vi "Host_17.vi"() -> ()   [LabVIEW 2017]
panel:
  in  "stop":bool
  out "Motor Speed":cluster{i32, dbl}[](graph)
  out "Armature Current":cluster{i32, dbl}[](graph)
  out "Feedback Load Torque 2":dbl
  out "Feedback Duty Cycle 2":dbl
  in  "Duty Cycle 2":dbl(slide) scale=0.0..100.0
  in  "Load Torque 2":dbl(slide) scale=-0.2..0.2
  in  "Data Update Speed (ms)":dbl
  in  "Website Button":bool
  in  "Doc Button":bool
  in  "Save Button":bool
  in  "Run Button":bool
  # "OPAL-RT Real Time Outputs"
  # "Microcontroller Inputs"
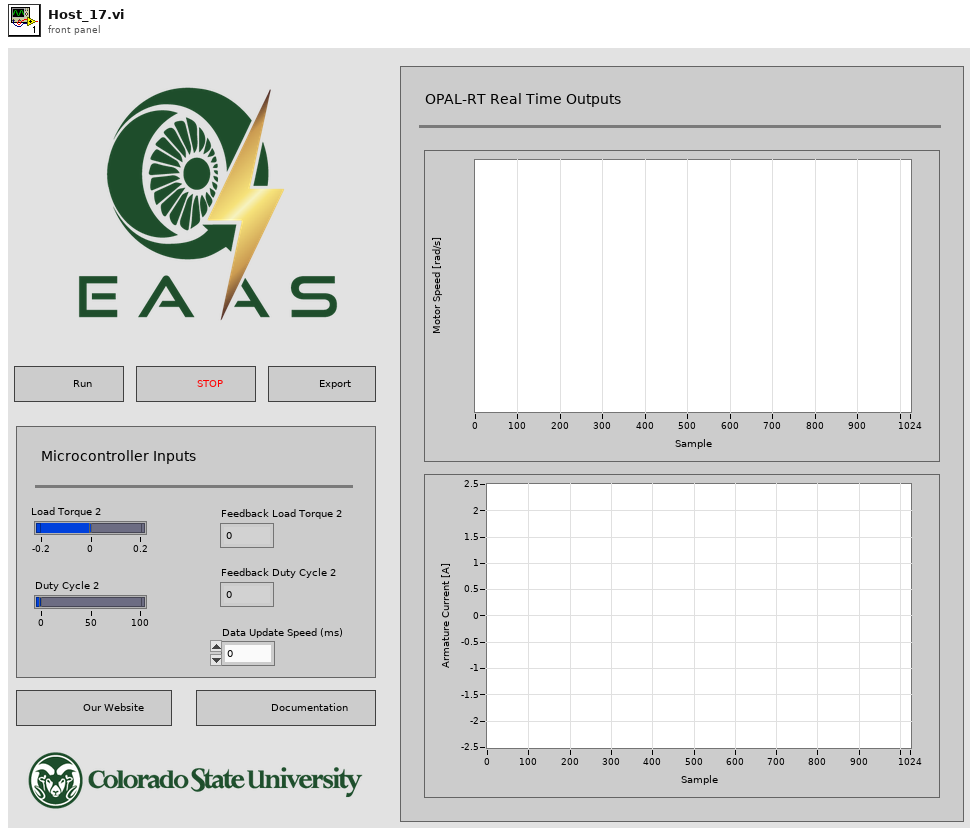
[diagram p1: front panel]
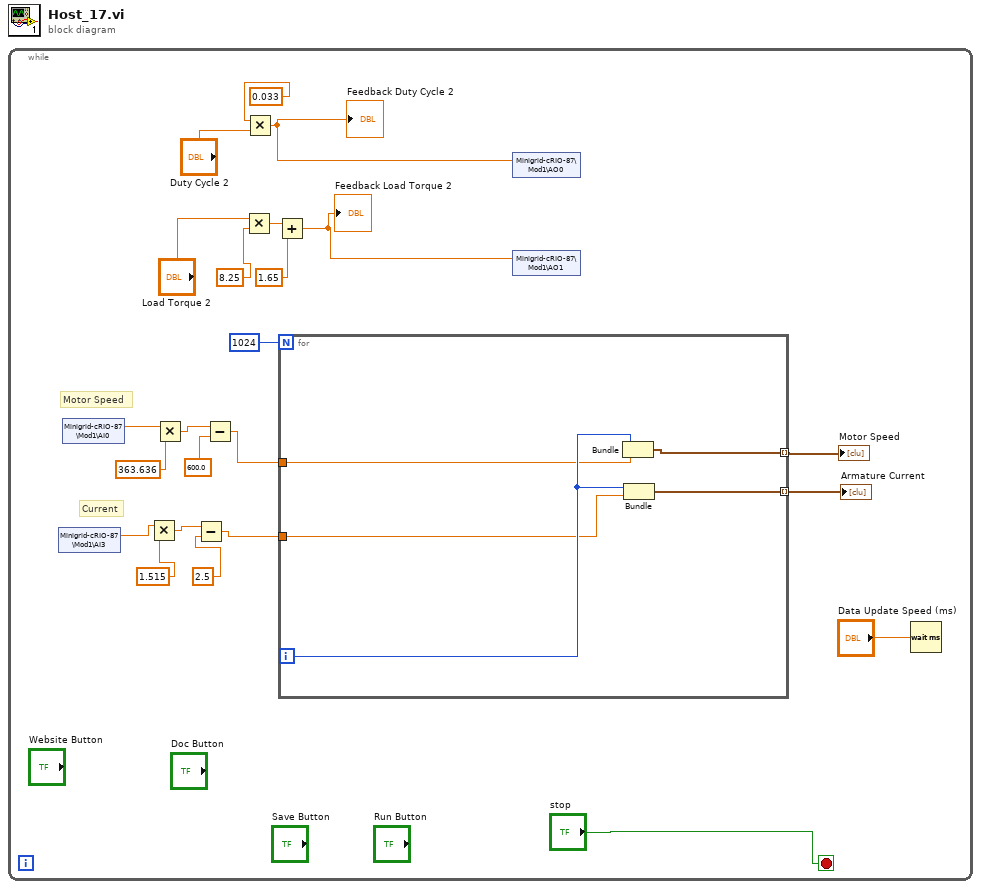
[diagram p0: block diagram]
diagram:
  n1 = while {
    stop <- "stop" stop-if-true
    # "Current"
    # "Motor Speed"
    n2 = shared-variable "Minigrid-cRIO-87\\Mod1\\AI3"() -> (w10:dbl)  [unwired: 1 in, 1 out]
    n3 = shared-variable "Minigrid-cRIO-87\\Mod1\\AI0"() -> (w9:dbl)  [unwired: 1 in, 1 out]
    n4 = Multiply(x=w10, y=1.515) -> (x*y=w8:dbl)
    n5 = Multiply(x=w9, y=363.636) -> (x*y=w7:dbl)
    n6 = Subtract(x=w8, y=2.5) -> (x-y=w2:dbl)
    n7 = Subtract(x=w7, y=600.0) -> (x-y=w1:dbl)
    n8 = Multiply(x="Load Torque 2", y=8.25) -> (x*y=w18:dbl)
    n9 = Multiply(x=0.033, y="Duty Cycle 2") -> (x*y=w15:dbl)
    "Feedback Duty Cycle 2" <- w15
    n10 = Add(x=w18, y=1.65) -> (x+y=w16:dbl)
    "Feedback Load Torque 2" <- w16
    n11 = for {
      N: 1024 -> [_]
      tunnel: [w28] -> w22 mode=indexing
      tunnel: [w27] -> w11 mode=indexing
      tunnel: w2 -> [w25]
      tunnel: w1 -> [w24]
      i -> [w26]
      n12 = Bundle(w26, w24) -> (w27:cluster{i32, dbl})  [unwired: 1 in]
      n13 = Bundle(w26, w25) -> (w28:cluster{i32, dbl})  [unwired: 1 in]
    }
    "Armature Current" <- w22
    "Motor Speed" <- w11
    n14 = shared-variable "Minigrid-cRIO-87\\Mod1\\AO0"(w15) -> ()  [unwired: 1 in, 1 out]
    n15 = shared-variable "Minigrid-cRIO-87\\Mod1\\AO1"(w16) -> ()  [unwired: 1 in, 1 out]
    n16 = Wait (ms)(milliseconds to wait="Data Update Speed (ms)") -> ()  [unwired: 1 out]
  }
